vi "DSF.Engine.Execution.Builder.Get Plugin Buffer.vi"(8 "error in (no error)":errorcluster, 9 "timeout ms (0)":i32 format="%d ms", 10 "plugin id":i32, 11 "Builder in":refnum<class "DSF.Engine.Execution.Builder.lvclass">) -> (0 "error out":errorcluster, 1 "timed out?":bool, 2 "Buffer":refnum<class "DSF.Engine.Memory.Buffer.lvclass">, 3 "Builder out":refnum<class "DSF.Engine.Execution.Builder.lvclass">)   [LabVIEW 2016, in "DSF.Engine.lvlib" / "DSF.Engine.Execution.Builder.lvclass"]
uses:
  Builder/DSF.Engine.Execution.Builder.lvclass
  Buffer/DSF.Engine.Memory.Buffer.lvclass
  Builder/DSF.Engine.Execution.Builder.lvclass/DSF.Engine.Execution.Builder.ctl
  BufferPool/DSF.Engine.Memory.BufferPool.lvclass/DSF.Engine.Memory.BufferPool.ctl
  DSF.Engine.Execution.Builder.Get Plugin Buffer Pools.vi
  Memory.BufferPool/DSF.Engine.Memory.BufferPool.Get Index FIFO.vi
  Memory.BufferPool/DSF.Engine.Memory.BufferPool.Get Buffers.vi
  BufferPool/DSF.Engine.Memory.BufferPool.lvclass
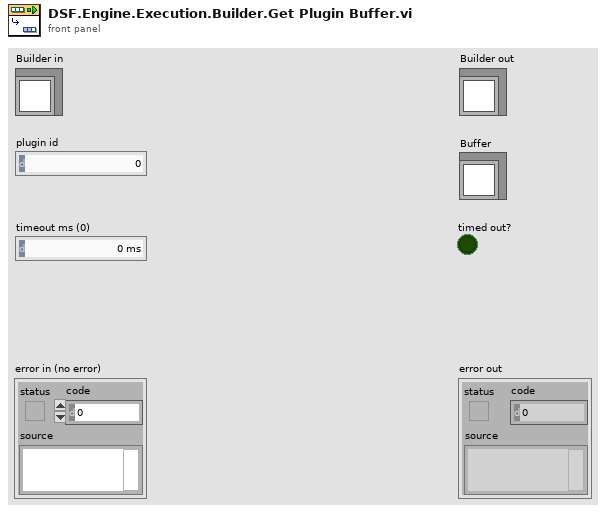
[diagram p1: front panel]
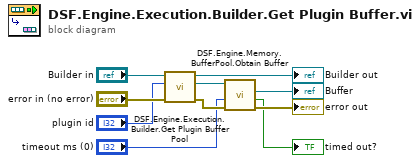
[diagram p0: block diagram]
diagram:
  n1 = call "DSF.Engine.Execution.Builder.Get Plugin Buffer Pool.vi"("error in (no error)"="error in (no error)", "plugin id"="plugin id", "Builder in"="Builder in") -> ("error out"=w6:errorcluster, "BufferPool"=w7:refnum<class "DSF.Engine.Memory.BufferPool.lvclass">, "Builder out"=→"Builder out":refnum<class "DSF.Engine.Execution.Builder.lvclass">)  [unwired: 6 in]
  n2 = call "DSF.Engine.Memory.BufferPool.Obtain Buffer.vi"("error in (no error)"=w6, "timeout ms (0)"="timeout ms (0)", "BufferPool in"=w7) -> ("error out"=→"error out":errorcluster, "timed out?"=→"timed out?":bool, "Buffer"=→"Buffer":refnum<class "DSF.Engine.Memory.Buffer.lvclass">)  [unwired: 5 in, 1 out]
